vi "StartPopup.vi"(7 "Popup":T1, 8 "error in (no error)":errorcluster, 11 "String parameter":string) -> (0 "error out":errorcluster)   [LabVIEW 2011]
uses:
  enumScreen.ctl
  050 - CONFIG/00 - ApplicationConfig/Ctrls/EnumFgvConfigCommand.ctl
  090 - ERRORS/Ctrls/EnumErrors.ctl
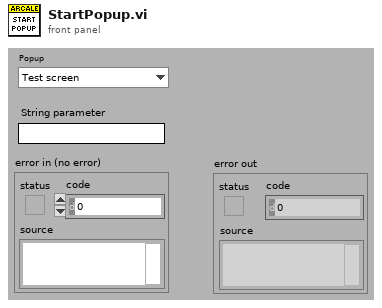
[diagram p1: front panel]
types:
  T1 = typedef "enumScreen.ctl" = enum16{"Test screen", "Ecran principal", "LOG", "Setup", "Popup : About", "Popup : View last message", "Popup : WebBrowser help", "Traduction", "Popup : DEBUG Process"}
  T2 = enum32{"Bad", "Idle", "Run top level", "Running"}
  T3 = typedef "EnumFgvConfigCommand.ctl" = enum16{"Load", "Get", "Set", "Save To Disk"}
  T4 = typedef "EnumErrors.ctl" = enum16{"VI non trouvé !", "Clé non trouvée", "Timeout", "Le VI tourne déjà", "Erreur de séparateur décimal", "Référence non trouvée"}
  T5 = typedef "ApplicationConfig.ctl" = cluster{"Data Path":path, "MessageHandlerConfig":T6, "Simulation":bool, "Dictionnary":string}
  T6 = typedef "MessageHandlerConfig.ctl" = cluster{"Max log files":u32, "Max messages per file":u32}
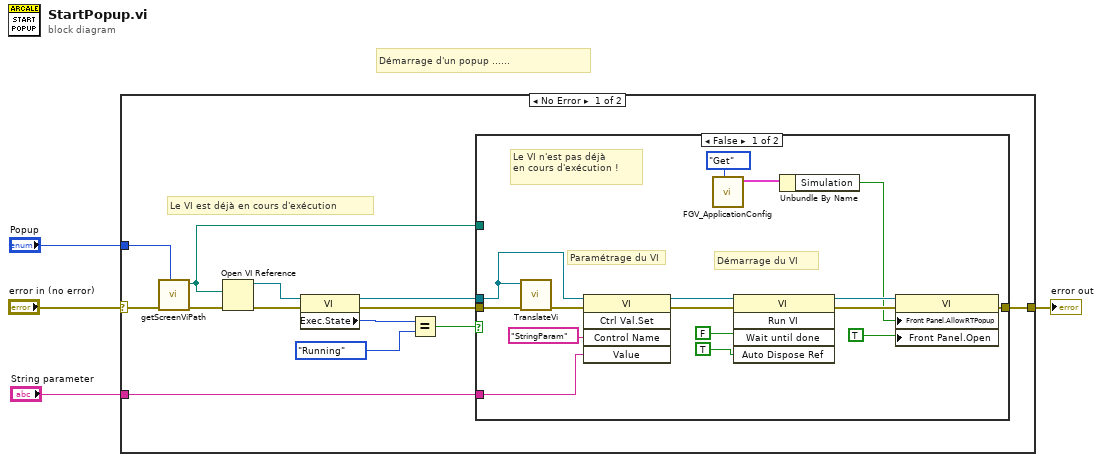
[diagram p0: block diagram]
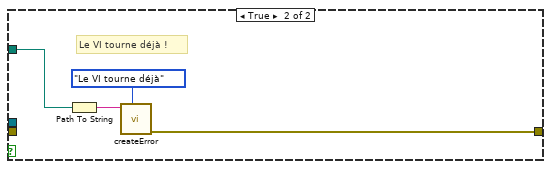
[diagram p2: hidden frame]
diagram:
  # "Démarrage d'un popup ......"
  n1 = case shown="No Error" "error in (no error)" {
    selector: "error in (no error)" -> [w8 w38]
    tunnel: [w10 w38] -> w4
    tunnel: "Popup" -> [w6 _]
    tunnel: "String parameter" -> [w5 _]
    frame No Error {
      # "Le VI est déjà en cours d'exécution"
      n2 = call "getScreenViPath.vi"("Enum Screen"=w6, "error in (no error)"=w8) -> ("error out"=w9:errorcluster, "Path"=w7:path)  [unwired: 1 in, 7 out]
      n3 = Open VI Reference(vi path=w7, error in (no error)=w9) -> (vi reference=w13:refnum<vi>, error out=w15:errorcluster)  [unwired: 1 in, 3 out]
      n4 = property class="VI"(reference=w13, error in=w15) -> (reference out=w12:refnum<vi>, error out=w14:errorcluster, "Exec.State"=w17:T2)
      n5 = Equal?(x=w17, y=T2."Running") -> (x = y?=w11:bool)
      n6 = case shown="False" w11 {
        tunnel: [w28 w37] -> w10
        tunnel: w14 -> [w22 _]
        tunnel: w12 -> [w23 _]
        tunnel: w7 -> [_ w35]
        tunnel: w5 -> [w24 _]
        frame False {
          # "Paramétrage du VI"
          # "Le VI n'est pas déjà\nen cours d'exécution !"
          # "Démarrage du VI"
          n7 = call "TranslateVi.vi"("error in (no error)"=w22, "VI ref"=w23) -> ("error out"=w21:errorcluster)  [unwired: 9 in]
          n8 = invoke class="VI" method="Ctrl Val.Set"(reference=w23, error in=w21, "Control Name"="StringParam", "Value"=w24) -> (reference out=w26:refnum<vi>, error out=w27:errorcluster)  [unwired: 1 in, 3 out]
          n9 = call "FGV_ApplicationConfig.vi"("Command"=EnumFgvConfigCommand."Get") -> ("ApplicationConfigOut"=w19:T5)  [unwired: 9 in, 1 out]
          n10 = invoke class="VI" method="Run VI"(reference=w26, error in=w27, "Wait until done"=FALSE ("Wait Until Done"), "Auto Dispose Ref"=TRUE ("Auto Dispose Reference")) -> (reference out=w30:refnum<vi>, error out=w29:errorcluster)  [unwired: 1 in, 3 out]
          n11 = Unbundle By Name(w19) -> ("Simulation"=w18:bool)
          n12 = property class="VI"(reference=w30, error in=w29, "Front Panel.AllowRTPopup"=w18, "Front Panel.Open"=TRUE ("Front Panel Window:Open")) -> (error out=w28:errorcluster)  [unwired: 1 out]
        }
        frame True {
          # "Le VI tourne déjà !"
          n13 = Path To String(path=w35) -> (string=w34:string)
          n14 = call "createError.vi"("ErrorCode"=EnumErrors."Le VI tourne déjà", "message"=w34) -> ("error out"=w37:errorcluster)  [unwired: 1 in, 8 out]
        }
      }
    }
    frame Error {
    }
  }
  "error out" <- w4
